vi "TestExec.PLC Wiggler Config.vi"(8 "error in (no error)":errorcluster, 11 "Config Folder":path=path "C:/MTE/Circle Test/Config") -> (0 "error out":errorcluster, 1 "PID":string, 2 "VID":string, 3 "Enabled":bool, 4 "Type":string)   [LabVIEW 2018]
uses:
  <vilib>/Utility/config.llb/Read Key (Boolean).vi
  <vilib>/Utility/config.llb/Read Key (String).vi
  <vilib>/Utility/config.llb/NI_LVConfig.lvlib
  <vilib>/KATE/Files/File Utils.lvlib
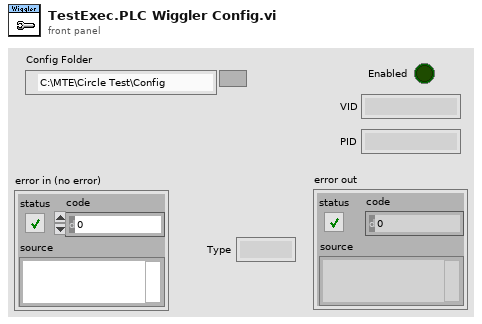
[diagram p1: front panel]
types:
  T1 = typedef "NI_LVConfig.lvlib/Config Data RefNum.ctl" = refnum<k1>
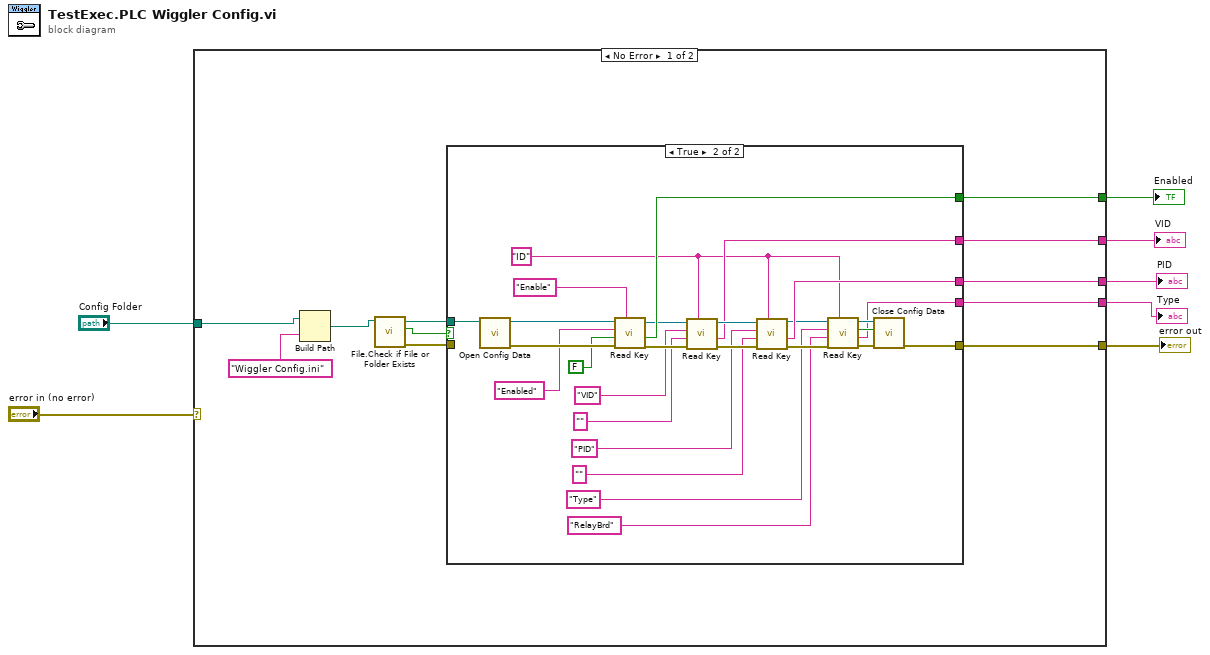
[diagram p0: block diagram]
diagram:
  n1 = case shown="No Error" "error in (no error)" {
    selector: "error in (no error)" -> [_ w46]
    tunnel: [w18 w46] -> w6
    tunnel: "Config Folder" -> [w17 _]
    tunnel: [w15 _] -> w4
    tunnel: [w10 _] -> w3
    tunnel: [w9 _] -> w2
    tunnel: [w8 _] -> w1
    frame No Error {
      n2 = Build Path(base path=w17, name or relative path="Wiggler Config.ini") -> (appended path=w14:path)
      n3 = call <vilib>:"File.Check if File or Folder Exists.vi"("Path"=w14) -> ("error out"=w11:errorcluster, "Exists"=w12:bool, "Dup Path"=w13:path)  [unwired: 6 in, 2 out]
      n4 = case shown="True" w12 {
        tunnel: [_ w43] -> w18
        tunnel: [_ w40] -> w15
        tunnel: w13 -> [_ w38]
        tunnel: w11 -> [_ _]
        tunnel: [_ w29] -> w10
        tunnel: [_ w28] -> w9
        tunnel: [_ w19] -> w8
        frame False {
        }
        frame True {
          w22 = "ID"
          n5 = call <vilib>:"Open Config Data.vi"("configuration file path"=w38) -> ("error out"=w45:errorcluster, "refnum"=w44:T1)  [unwired: 8 in, 1 out]
          n6 = call-poly <vilib>:"Read Key.vi"("section"="Enable", "error in (no error)"=w45, "default value"=FALSE, "key"="Enabled", "refnum"=w44) -> ("error out"=w34:errorcluster, "value"=w40:bool, "refnum out"=w37:T1)  [unwired: 3 in, 1 out]
          n7 = call-poly <vilib>:"Read Key.vi"("section"=w22, "error in (no error)"=w34, "default value"="", "key"="VID", "refnum"=w37) -> ("error out"=w35:errorcluster, "value"=w29:string, "refnum out"=w36:T1)  [unwired: 3 in, 1 out]
          n8 = call-poly <vilib>:"Read Key.vi"("section"=w22, "error in (no error)"=w35, "default value"="", "key"="PID", "refnum"=w36) -> ("error out"=w23:errorcluster, "value"=w28:string, "refnum out"=w24:T1)  [unwired: 3 in, 1 out]
          n9 = call-poly <vilib>:"Read Key.vi"("section"=w22, "error in (no error)"=w23, "default value"="RelayBrd", "key"="Type", "refnum"=w24) -> ("error out"=w27:errorcluster, "value"=w19:string, "found?"=w26:bool, "refnum out"=w25:T1)  [unwired: 3 in]
          n10 = call <vilib>:"Close Config Data.vi"("error in (no error)"=w27, "write file if changed (T)"=w26, "refnum"=w25) -> ("error out"=w43:errorcluster)  [unwired: 7 in, 1 out]
        }
      }
    }
    frame Error {
    }
  }
  "error out" <- w6
  "Enabled" <- w4
  "VID" <- w3
  "PID" <- w2
  "Type" <- w1
